vi "Create Network.vi"(0 "#Inputs":u32, 1 "Classification(F)/Regression(T)":bool, 5 "#Outputs":u32, 11 "Error In":errorcluster) -> (4 "Neural Network":refnum<class "Neural Network.lvclass">, 15 "Error Out":errorcluster)   [LabVIEW 2015, in "Neural Network.lvclass"]
doc: "Create a general purpose neural network with 2 hidden layers. This means that the network has 4 layers: input, hidden1, hidden2 and output. Network implements scaling of input and output values to and from the range of 0.2 to 0.8. This makes the unipolar sigmoidal activation function of the neurons most effective.\n\n<b>Classification(F)/Regression(T)</b> - If the output values that you want to get from the network are not bound by max and min values you should set the this input to True. This setting allows the network to output effectivly beyond the range of values that you teach it with, by setting the last layer to be linear instead of unipolar sigmoidal."
uses:
  Neural Network.lvclass
  <vilib>/ErrorRing/Error Ring.xnode
  <vilib>/Utility/error.llb/Error Cluster From Error Code.vi
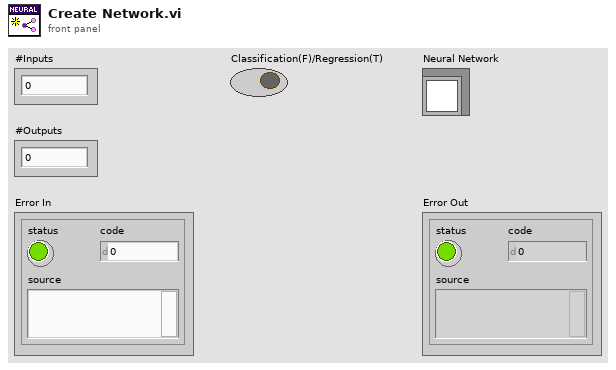
[diagram p1: front panel]
types:
  T1 = typedef "Neural Network.lvclass/2D Array.ctl" = cluster{"2D Array":sgl[][]}
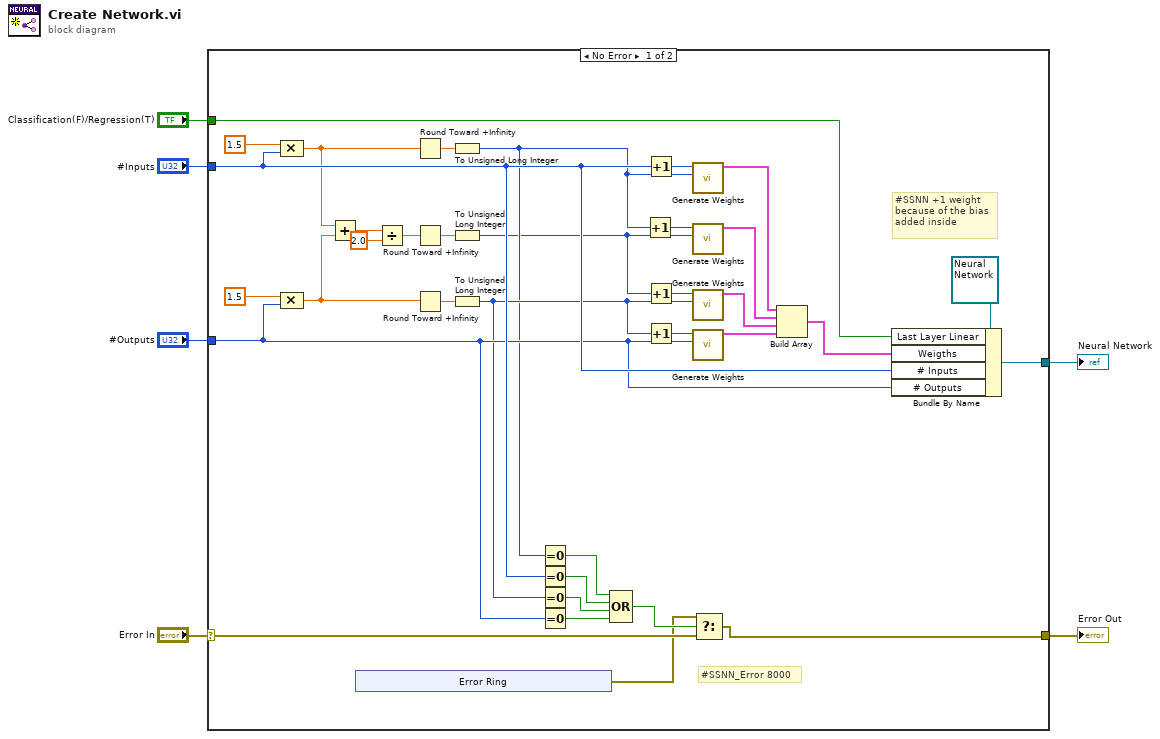
[diagram p0: block diagram]
diagram:
  n1 = case shown="No Error" "Error In" {
    selector: "Error In" -> [w26 w47]
    tunnel: [w41 _] -> w6
    tunnel: "Classification(F)/Regression(T)" -> [w39 _]
    tunnel: "#Outputs" -> [w19 _]
    tunnel: "#Inputs" -> [w23 _]
    tunnel: [w25 w47] -> w1
    frame No Error {
      # "#SSNN_Error 8000"
      # "#SSNN +1 weight\nbecause of the bias\nadded inside"
      n2 = Compound Arithmetic op=MULTIPLY(1.5 ("value"), w23) -> (w15:dbl)
      n3 = Compound Arithmetic op=MULTIPLY(1.5 ("value"), w19) -> (w17:dbl)
      n4 = Add(x=w15, y=w17) -> (x+y=w14:dbl)
      n5 = xnode "Error Ring"() -> ("error out"=w24:errorcluster)
      n6 = Divide(x=w14, y=2.0) -> (x/y=w11:dbl)
      n7 = Round Toward +Infinity(x=w15) -> (ceil(x): smallest int >= x=w22:dbl)
      n8 = Round Toward +Infinity(x=w11) -> (ceil(x): smallest int >= x=w12:dbl)
      n9 = Round Toward +Infinity(x=w17) -> (ceil(x): smallest int >= x=w21:dbl)
      n10 = To Unsigned Long Integer(number=w22) -> (unsigned 32bit integer=w10:u32)
      n11 = To Unsigned Long Integer(number=w12) -> (unsigned 32bit integer=w8:u32)
      n12 = To Unsigned Long Integer(number=w21) -> (unsigned 32bit integer=w18:u32)
      n13 = Equal To 0?(x=w10) -> (x = 0?=w27:bool)
      n14 = Equal To 0?(x=w23) -> (x = 0?=w29:bool)
      n15 = Equal To 0?(x=w18) -> (x = 0?=w30:bool)
      n16 = Equal To 0?(x=w19) -> (x = 0?=w31:bool)
      n17 = Compound Arithmetic op=OR(w27, w29, w30, w31) -> (w28:bool)
      n18 = Increment(x=w10) -> (x+1=w9:u32)
      n19 = Increment(x=w23) -> (x+1=w36:u32)
      n20 = Increment(x=w8) -> (x+1=w38:u32)
      n21 = Increment(x=w18) -> (x+1=w37:u32)
      n22 = call "Generate Weights.vi"("Neurons"=w10, "Inputs"=w36) -> ("Layer Weights"=w34:T1)  [unwired: 9 in]
      n23 = call "Generate Weights.vi"("Neurons"=w8, "Inputs"=w9) -> ("Layer Weights"=w7:T1)  [unwired: 9 in]
      n24 = call "Generate Weights.vi"("Neurons"=w18, "Inputs"=w38) -> ("Layer Weights"=w33:T1)  [unwired: 9 in]
      n25 = call "Generate Weights.vi"("Neurons"=w19, "Inputs"=w37) -> ("Layer Weights"=w32:T1)  [unwired: 9 in]
      n26 = Select(t=w24, s=w28, f=w26) -> (s? t:f=w25:errorcluster)
      n27 = Build Array(w34, w7, w33, w32) -> (w35:T1[])
      n28 = Bundle By Name(cluster=refnum<class "Neural Network.lvclass"> refnum ("Neural Network"), "Last Layer Linear"=w39, "Weigths"=w35, "# Inputs"=w23, "# Outputs"=w19) -> (w41:refnum<class "Neural Network.lvclass">)
    }
    frame Error {
    }
  }
  "Neural Network" <- w6
  "Error Out" <- w1
